vi "FindHawkeyePath.vi"(8 "error in (no error)":errorcluster, 10 "Workspace Path":path, 11 "Library/Class Name":string) -> (0 "error out":errorcluster, 2 "Found?":bool, 3 "Hawkeye Path":path)   [LabVIEW 2019, in "Hawkeye.lvlib"]
uses:
  <userlib>/_OpenG.lib/file/file.llb/Valid Path - Traditional__ogtk.vi
  <userlib>/_OpenG.lib/file/file.llb/File Exists - Scalar__ogtk.vi
  Hawkeye.lvlib
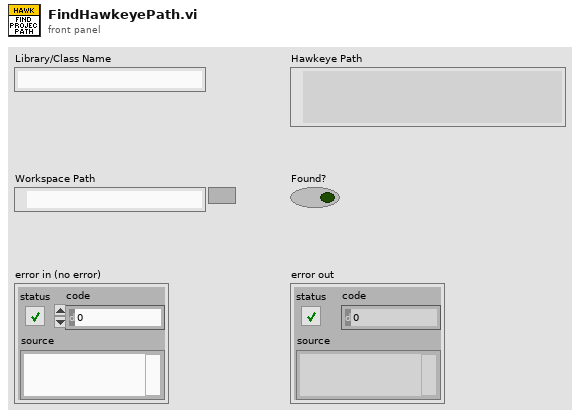
[diagram p1: front panel]
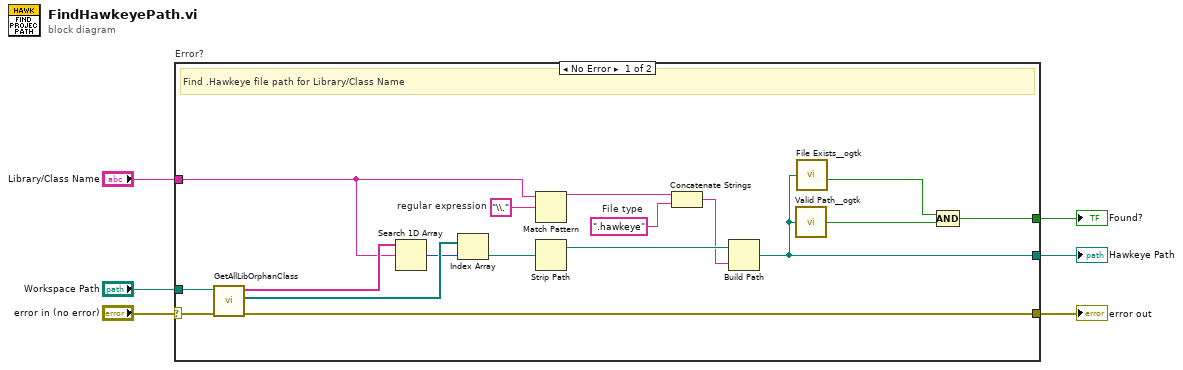
[diagram p0: block diagram]
diagram:
  n1 = case "Error?" shown="No Error" "error in (no error)" {
    selector: "error in (no error)" -> [w22 w24]
    tunnel: "Library/Class Name" -> [w17 _]
    tunnel: "Workspace Path" -> [w12 _]
    tunnel: [w11 _] -> w3
    tunnel: [w8 _] -> w2
    tunnel: [w7 w24] -> w1
    frame No Error {
      w14 = ".hawkeye"  # File type
      w16 = "\\."  # regular expression
      # "Find .Hawkeye file path for Library/Class Name"
      n2 = call "GetAllLibOrphanClass.vi"("error in (no error)"=w22, "Workspace Path"=w12) -> ("error out"=w7:errorcluster, "Lib / Class Path []"=w21:path[], "Lib / Class Name []"=w23:string[])  [unwired: 7 in]
      n3 = Search 1D Array(1D array=w23, element=w17) -> (index of element=w20:i32)  [unwired: 1 in]
      n4 = Index Array(array=w21, index=w20) -> (element=w19:path)
      n5 = Match Pattern(string=w17, regular expression=w16) -> (before substring=w15:string)  [unwired: 1 in, 3 out]
      n6 = Strip Path(path=w19) -> (stripped path=w18:path)  [unwired: 1 out]
      n7 = Concatenate Strings(w15, w14) -> (w13:string)
      n8 = Build Path(base path=w18, name or relative path=w13) -> (appended path=w11:path)
      n9 = call-poly <userlib>:"Valid Path__ogtk.vi"("path"=w11) -> ("valid"=w9:bool)
      n10 = call-poly <userlib>:"File Exists__ogtk.vi"("file path"=w11) -> ("exists"=w10:bool)  [unwired: 6 in, 1 out]
      n11 = Compound Arithmetic op=AND(w10, w9) -> (w8:bool)
    }
    frame Error {
      # "Error"
    }
  }
  "Hawkeye Path" <- w3
  "Found?" <- w2
  "error out" <- w1
